vi "RP Transmit Data TCP.vi"(8 "Error In":errorcluster, 10 "Data":u32[](array[numeric]), 11 "connection ID":refnum<k5>) -> (0 "Error Out":errorcluster, 3 "connection ID out":refnum<k5>)   [LabVIEW 2016]
uses:
  RP Command.ctl
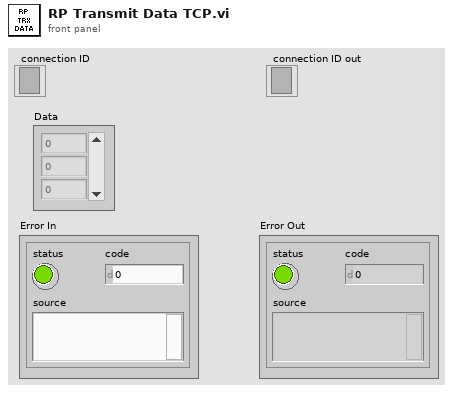
[diagram p1: front panel]
types:
  T1 = typedef "RP Command.ctl" = enum16{"Reset", "Read IDN", "Stop server", "Get status", "Get temperature", "Connect client", "Arm", "Software trigger", "Get whole buffer", "Get chunk", "System call", "Get config", "Set config", "Recieve data", "Play pattern", "Transmit data"}
  T2 = enum16{"big-endian, network order", "native, host order", "little-endian"}
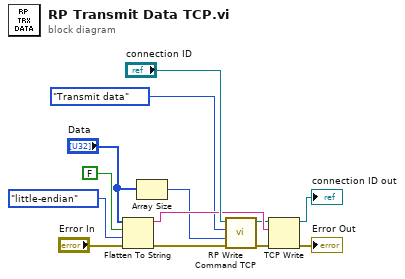
[diagram p0: block diagram]
diagram:
  n1 = Flatten To String(anything="Data", prepend array or string size? (T)=FALSE, byte order (0:big-endian, network order)=T2."little-endian", error in (no error)="Error In") -> (data string=w10:string, error out=w5:errorcluster)  [unwired: 1 out]
  n2 = Array Size(array="Data") -> (size(s)=w1:i32)
  n3 = call "RP Write Command TCP.vi"("Error In"=w5, "Command payload"=w1, "Command number"=RP_Command."Transmit data", "connection ID"="connection ID") -> ("Error Out"=w4:errorcluster, "connection ID out"=w9:refnum<k5>)  [unwired: 5 in, 1 out]
  n4 = TCP Write(connection ID=w9, data in=w10, error in (no error)=w4) -> (connection ID out=→"connection ID out":refnum<k5>, error out=→"Error Out":errorcluster)  [unwired: 1 in, 1 out]
